vi "Calculate Measurement Query.vi"(8 "error in":errorcluster, 10 "Calculation Channel":i32(ring) items=["Calc Channel 1", "Calc Channel 2", "Calc Channel 3", "Calc Channel 4"], 11 "Instrument Handle In":i32) -> (0 "error out":errorcluster, 1 "Type":i32, 2 "Source":i32, 3 "Instrument Handle Out":i32)   [LabVIEW 8.6, in "ZTScopeM.lvlib"]
doc: "Query the measurement trending configuration of the selected calculation channel."
uses:
  ZTScopeM.lvlib
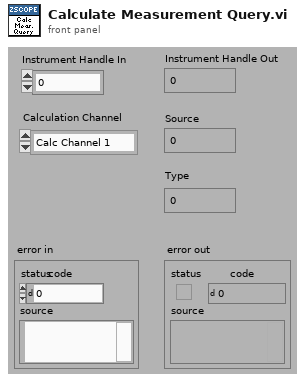
[diagram p1: front panel]
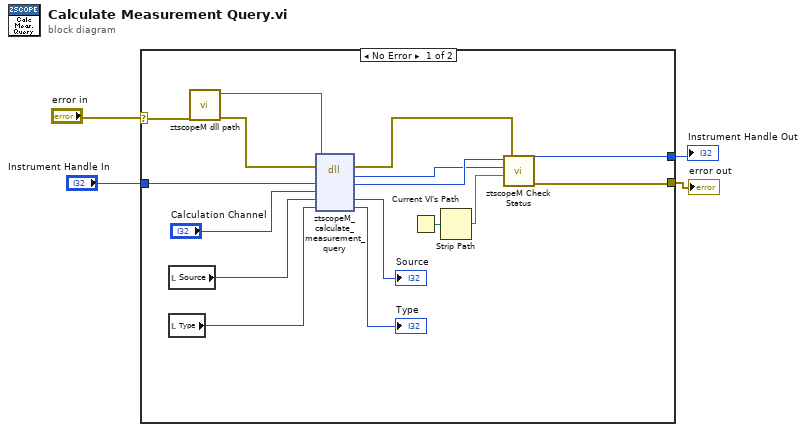
[diagram p0: block diagram]
diagram:
  n1 = case shown="No Error" "error in" {
    selector: "error in" -> [w8 w22]
    tunnel: [w10 w22] -> w2
    tunnel: "Instrument Handle In" -> [w20 w21]
    tunnel: [w9 w21] -> w1
    frame #0 {
      n2 = local read "Source"() -> (w18:i32)
      n3 = local read "Type"() -> (w16:i32)
      n4 = call "ztscopeM dll path.vi"("error in (no error)"=w8) -> ("error out"=w6:errorcluster, "<instrument>.dll path"=w7:path)  [unwired: 9 in]
      n5 = dll-call lib="C:/Program Files (x86)/National Instruments/LabVIEW 2013/instr.lib/ztscopem/ztscopeM.dll" fn="ztscopeM_calculate_measurement_query"(path in=w7, error in=w6, "instrumentHandle"=w20, "calculationChannel"="Calculation Channel", "source"=w18, "type"=w16) -> (error out=w5:errorcluster, w11:i32, "instrumentHandle"=w12:i32, "source"=→"Source":i32, "type"=→"Type":i32)  [unwired: 2 in, 1 out]
      n6 = Current VI's Path() -> (path=w14:path)
      n7 = Strip Path(path=w14) -> (name=w13:string)  [unwired: 1 out]
      n8 = call "ztscopeM Check Status.vi"("error in"=w5, "name of VI"=w13, "status (return code)"=w11, "instrument handle in"=w12) -> ("error out"=w10:errorcluster, "instrument handle out"=w9:i32)  [unwired: 2 in]
    }
    frame #1 {
    }
  }
  "Instrument Handle Out" <- w1
  "error out" <- w2
